vi "Init.vi"(8 "error in (no error)":errorcluster, 11 "UserPreferencesFileManager in":refnum<class "User Preferences File.lvclass">) -> (0 "error out":errorcluster, 3 "UserPreferencesFileManager out":refnum<class "User Preferences File.lvclass">)   [LabVIEW 2020, in "User Preferences File.lvclass"]
doc: "Initialize the file manager with default file names and locations for the given operating system. This VI does not create the file or load it."
uses:
  User Preferences File.lvclass
  User Preferences File.lvclass/User Preferences File.ctl
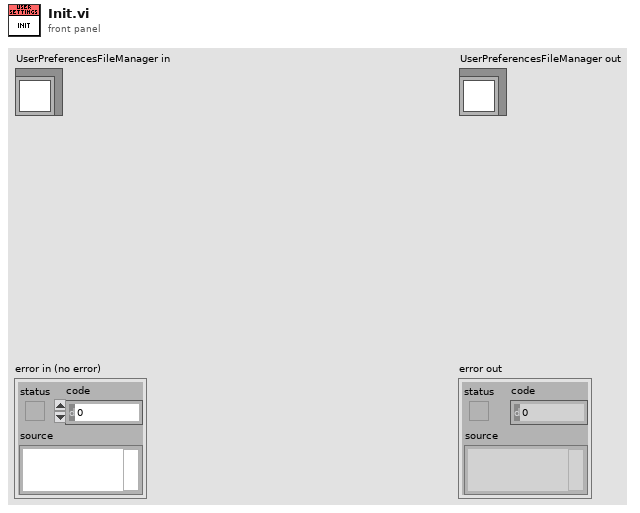
[diagram p1: front panel]
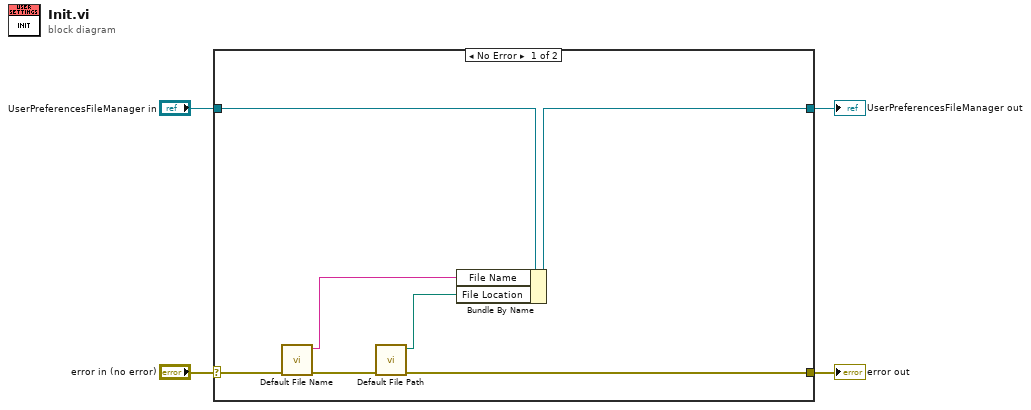
[diagram p0: block diagram]
diagram:
  n1 = case shown="No Error" "error in (no error)" {
    selector: "error in (no error)" -> [w11 w13]
    tunnel: [w5 w13] -> w3
    tunnel: [w8 w12] -> w1
    tunnel: "UserPreferencesFileManager in" -> [w9 w12]
    frame No Error {
      n2 = call "Default File Name.vi"("error in (no error)"=w11) -> ("error out"=w10:errorcluster, "Default File Name"=w7:string)  [unwired: 9 in]
      n3 = call "Default File Path.vi"("error in (no error)"=w10) -> ("error out"=w5:errorcluster, "Default File Path"=w6:path)  [unwired: 9 in]
      n4 = Bundle By Name(cluster=w9, "File Name"=w7, "File Location"=w6) -> (w8:refnum<class "User Preferences File.lvclass">)
    }
    frame Error {
    }
  }
  "error out" <- w3
  "UserPreferencesFileManager out" <- w1
